vi "GetFileManagerDeviceConstants.vi"(9 "device":T2, 10 "key values":T13[](array[typedef]), 11 "config":T1) -> (3 "config out":T1)   [LabVIEW 2017]
uses:
  <vilib>/addons/InsightCM/MessageBus/Base/controls/SectionKeyValues.ctl
  <vilib>/addons/InsightCM/MessageBus/Base/controls/KeyValuePair.ctl
  <vilib>/addons/InsightCM/MessageBus/Base/controls/R2_Device.ctl
  <vilib>/addons/InsightCM/MessageBus/Base/controls/DeviceState.ctl
  <vilib>/addons/InsightCM/MessageBus/Base/controls/R2_DataGroup.ctl
  <vilib>/addons/InsightCM/MessageBus/Base/controls/OperatingState.ctl
  <vilib>/addons/InsightCM/MessageBus/Base/controls/Trigger.ctl
  <vilib>/addons/InsightCM/MessageBus/Base/controls/Condition.ctl
  <vilib>/addons/InsightCM/MessageBus/Base/controls/BurstModeTrigger.ctl
  <vilib>/addons/InsightCM/MessageBus/Base/controls/DeviceSensorGroup.ctl
  <vilib>/addons/InsightCM/MessageBus/Base/controls/Endpoint.ctl
  <vilib>/addons/InsightCM/MessageBus/Base/controls/WirelessChannel.ctl
  <vilib>/addons/InsightCM/Devices/Shared/Common/FileManager/controls/config.ctl
  <vilib>/addons/InsightCM/Utilities/PropertyHelpers/PropertyHelpers.lvlib
  <vilib>/addons/InsightCM/Devices/Shared/Common/FileManager/FileManager.lvlib
panel:
  out "backlog extra large files":bool
  out "backlog file batch size":i32
  out "backlog trend points":bool
  out "backlog stream trend points":bool
  out "clean up file folders interval (sec)":dbl
  out "backlog file interval (sec)":dbl
  out "max files in memory":i32
  out "min drive free space":i32
  out "manage drive interval (sec)":dbl
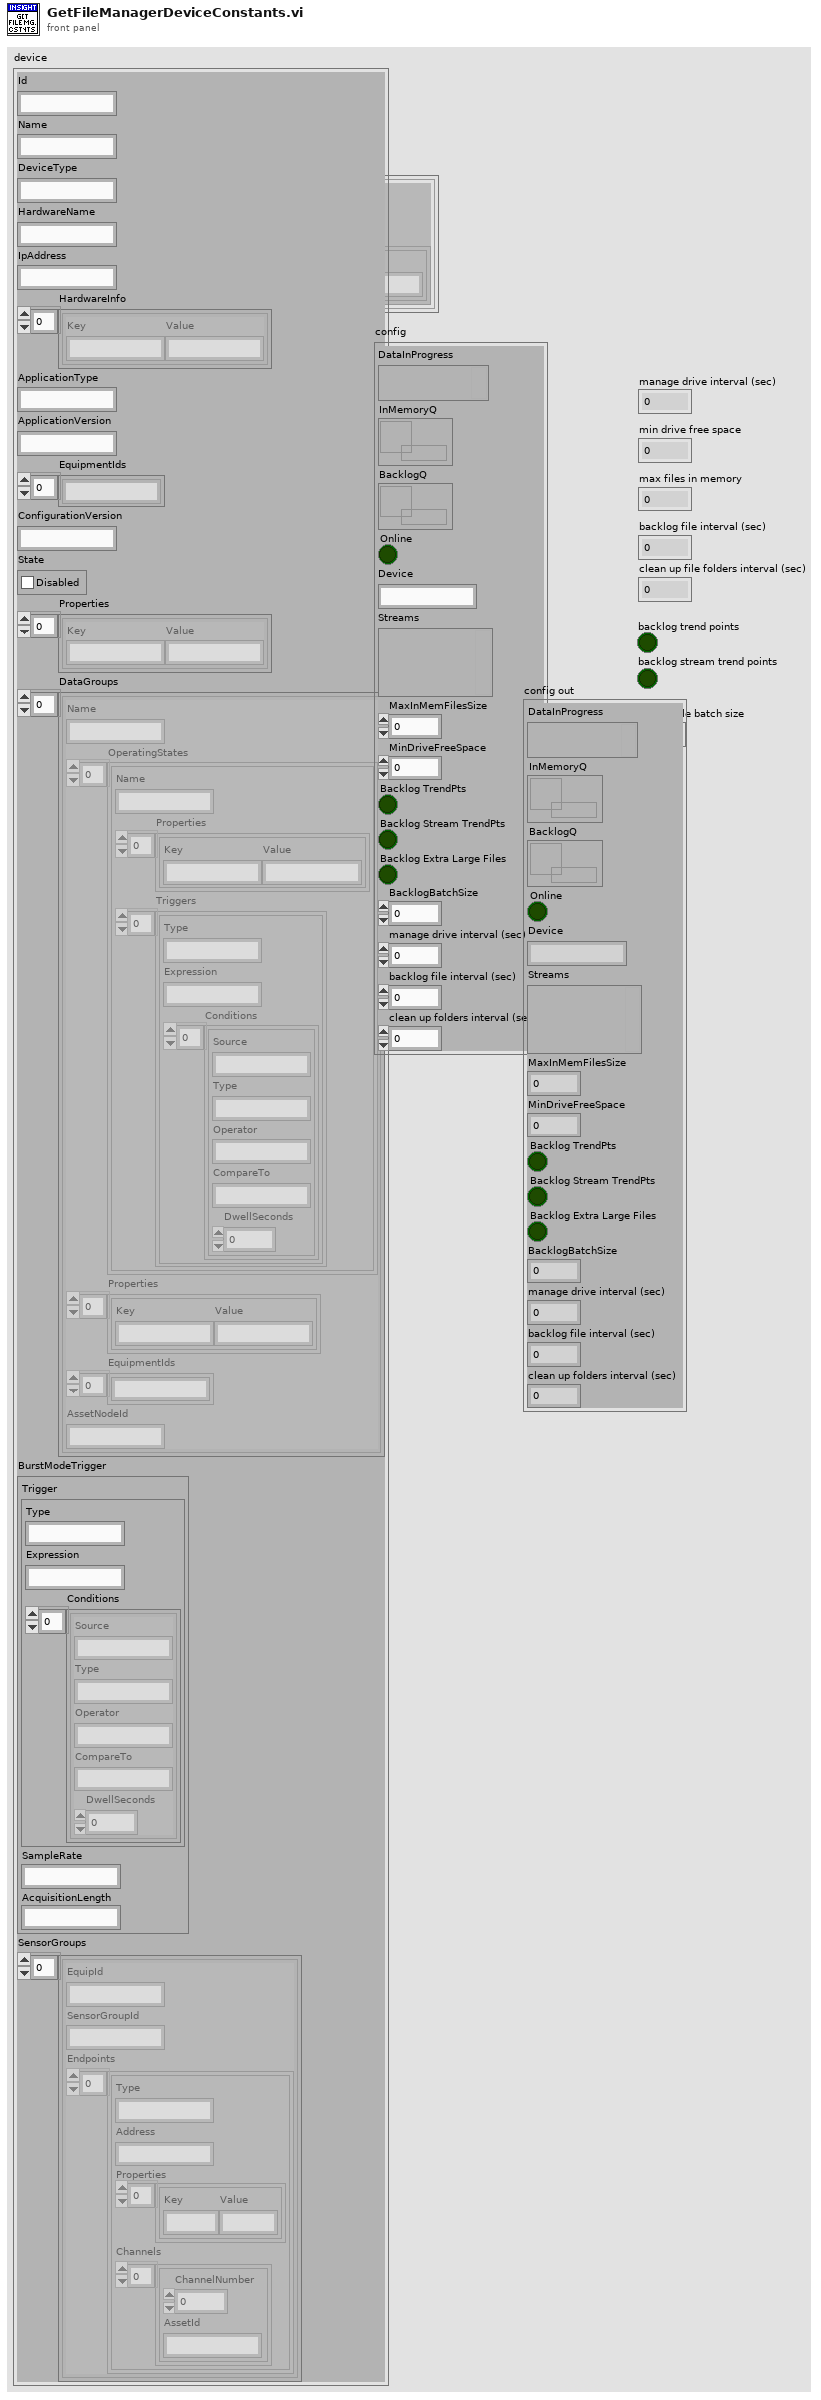
[diagram p1: front panel]
types:
  T1 = typedef "FileManager.lvlib/config.ctl" = cluster{"DataInProgress":variant, "InMemoryQ":refnum<queue>, "BacklogQ":refnum<queue>, "Online":bool, "Device":string, "Streams":variant, "MaxInMemFilesSize":i32, "MinDriveFreeSpace":i32, "Backlog TrendPts":bool, "Backlog Stream TrendPts":bool, "Backlog Extra Large Files":bool, "BacklogBatchSize":i32, "manage drive interval (sec)":dbl, "backlog file interval (sec)":dbl, "clean up folders interval (sec)":dbl}
  T2 = typedef "R2_Device.ctl" = cluster{"Id":string, "Name":string, "DeviceType":string, "HardwareName":string, "IpAddress":string, "HardwareInfo":T3[], "ApplicationType":string, "ApplicationVersion":string, "EquipmentIds":string[], "ConfigurationVersion":string, "State":T4, "Properties":T3[], "DataGroups":T5[], "BurstModeTrigger":T9, "SensorGroups":T10[]}
  T3 = typedef "KeyValuePair.ctl" = cluster{"Key":string, "Value":string}
  T4 = typedef "DeviceState.ctl" = cluster{"Disabled":bool}
  T5 = typedef "R2_DataGroup.ctl" = cluster{"Name":string, "OperatingStates":T6[], "Properties":T3[], "EquipmentIds":string[], "AssetNodeId":string}
  T6 = typedef "OperatingState.ctl" = cluster{"Name":string, "Properties":T3[], "Triggers":T7[]}
  T7 = typedef "Trigger.ctl" = cluster{"Type":string, "Expression":string, "Conditions":T8[]}
  T8 = typedef "Condition.ctl" = cluster{"Source":string, "Type":string, "Operator":string, "CompareTo":string, "DwellSeconds":dbl}
  T9 = typedef "BurstModeTrigger.ctl" = cluster{"Trigger":T7, "SampleRate":string, "AcquisitionLength":string}
  T10 = typedef "DeviceSensorGroup.ctl" = cluster{"EquipId":string, "SensorGroupId":string, "Endpoints":T11[]}
  T11 = typedef "Endpoint.ctl" = cluster{"Type":string, "Address":string, "Properties":T3[], "Channels":T12[]}
  T12 = typedef "WirelessChannel.ctl" = cluster{"ChannelNumber":i32, "AssetId":string}
  T13 = typedef "SectionKeyValues.ctl" = cluster{"Section":string, "KeyValues":T3[]}
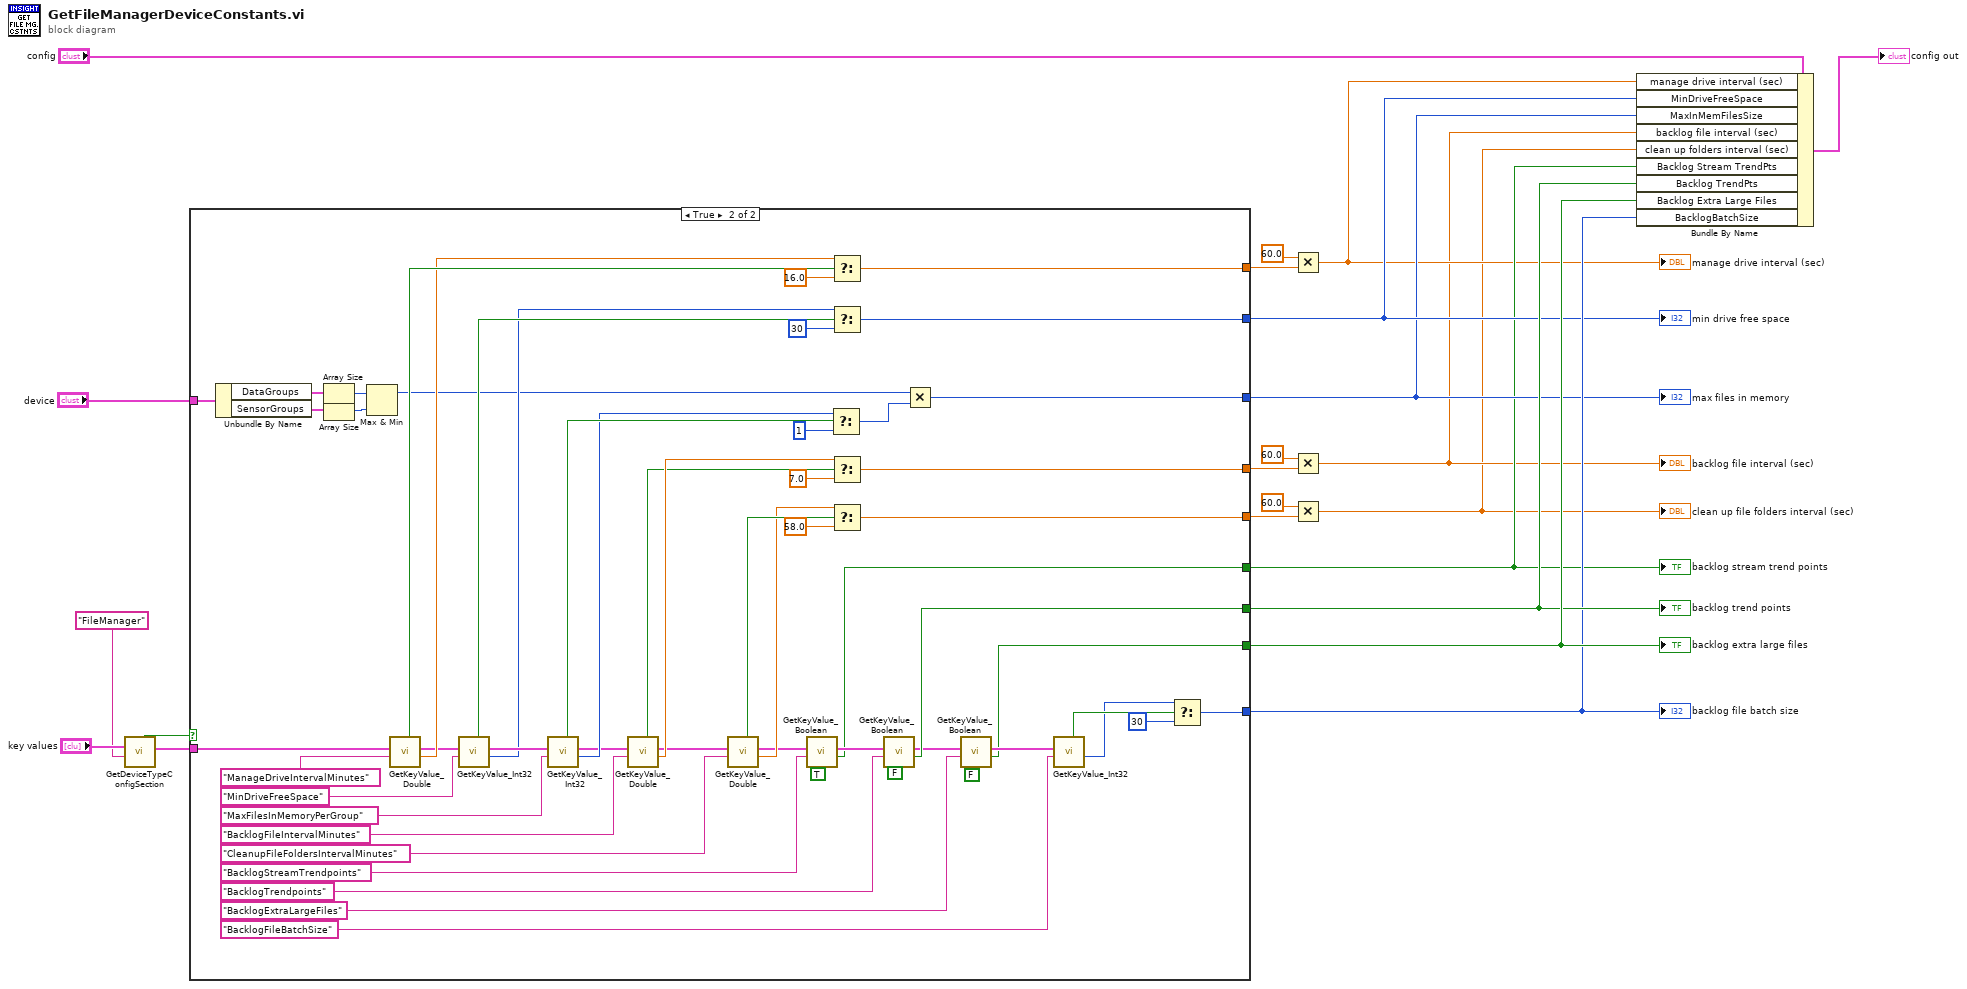
[diagram p0: block diagram]
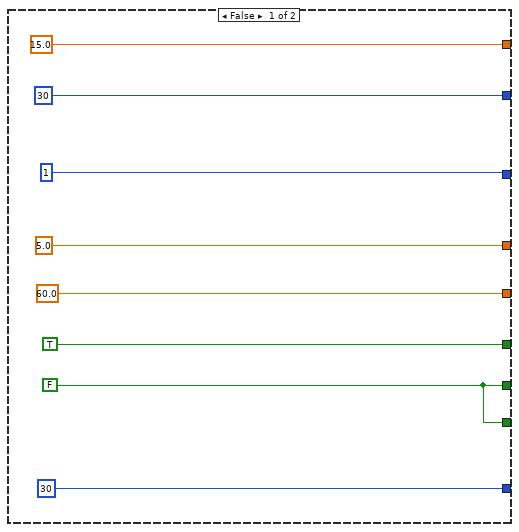
[diagram p2: hidden frame]
diagram:
  n1 = call <vilib>:"GetDeviceTypeConfigSection.vi"("key"="FileManager", "key values"="key values") -> ("key value pairs out"=w20:T3[], "found"=w21:bool)  [unwired: 8 in]
  n2 = case shown="True" w21 {
    tunnel: w20 -> [_ w85]
    tunnel: [15.0 ("f") w71] -> w18
    tunnel: [30 ("f") w70] -> w6
    tunnel: [1 ("f") w59] -> w5
    tunnel: [5.0 ("f") w66] -> w17
    tunnel: "device" -> [_ w62]
    tunnel: [60.0 ("f") w53] -> w12
    tunnel: [TRUE ("value") w40] -> w4
    tunnel: [w23 w42] -> w8
    tunnel: [30 ("f") w44] -> w7
    tunnel: [w23 w36] -> w9
    frame False {
      w23 = FALSE ("value")
    }
    frame True {
      n3 = Unbundle By Name(w62) -> ("DataGroups"=w61:T5[], "SensorGroups"=w34:T10[])
      n4 = Array Size(array=w61) -> (size(s)=w32:i32)
      n5 = Array Size(array=w34) -> (size(s)=w33:i32)
      n6 = Max & Min(x=w32, y=w33) -> (max(x,y)=w31:i32)  [unwired: 1 out]
      n7 = call <vilib>:"GetKeyValue_Double.vi"("key"="ManageDriveIntervalMinutes" ("Key"), "key value pairs"=w85) -> ("value"=w83:dbl, "key value pairs out"=w81:T3[], "found"=w84:bool)  [unwired: 7 in]
      n8 = call <vilib>:"GetKeyValue_Int32.vi"("key"="MinDriveFreeSpace" ("Key"), "key value pairs"=w81) -> ("value"=w76:i32, "key value pairs out"=w80:T3[], "found"=w78:bool)  [unwired: 7 in]
      n9 = call <vilib>:"GetKeyValue_Int32.vi"("key"="MaxFilesInMemoryPerGroup", "key value pairs"=w80) -> ("value"=w75:i32, "key value pairs out"=w67:T3[], "found"=w77:bool)  [unwired: 7 in]
      n10 = call <vilib>:"GetKeyValue_Double.vi"("key"="BacklogFileIntervalMinutes" ("Key"), "key value pairs"=w67) -> ("value"=w64:dbl, "key value pairs out"=w55:T3[], "found"=w63:bool)  [unwired: 7 in]
      n11 = call <vilib>:"GetKeyValue_Double.vi"("key"="CleanupFileFoldersIntervalMinutes" ("Key"), "key value pairs"=w55) -> ("value"=w57:dbl, "key value pairs out"=w52:T3[], "found"=w58:bool)  [unwired: 7 in]
      n12 = call <vilib>:"GetKeyValue_Boolean.vi"("default value"=TRUE, "key"="BacklogStreamTrendpoints", "key value pairs"=w52) -> ("value"=w40:bool, "key value pairs out"=w50:T3[])  [unwired: 6 in, 1 out]
      n13 = Select(t=w75, s=w77, f=1) -> (s? t:f=w60:i32)
      n14 = Select(t=w83, s=w84, f=16.0) -> (s? t:f=w71:dbl)
      n15 = Select(t=w76, s=w78, f=30) -> (s? t:f=w70:i32)
      n16 = Select(t=w64, s=w63, f=7.0) -> (s? t:f=w66:dbl)
      n17 = Select(t=w57, s=w58, f=58.0) -> (s? t:f=w53:dbl)
      n18 = call <vilib>:"GetKeyValue_Boolean.vi"("default value"=FALSE, "key"="BacklogTrendpoints", "key value pairs"=w50) -> ("value"=w42:bool, "key value pairs out"=w39:T3[])  [unwired: 6 in, 1 out]
      n19 = Multiply(x=w31, y=w60) -> (x*y=w59:i32)
      n20 = call <vilib>:"GetKeyValue_Boolean.vi"("default value"=FALSE, "key"="BacklogExtraLargeFiles", "key value pairs"=w39) -> ("value"=w36:bool, "key value pairs out"=w38:T3[])  [unwired: 6 in, 1 out]
      n21 = call <vilib>:"GetKeyValue_Int32.vi"("key"="BacklogFileBatchSize", "key value pairs"=w38) -> ("value"=w46:i32, "found"=w47:bool)  [unwired: 7 in, 1 out]
      n22 = Select(t=w46, s=w47, f=30) -> (s? t:f=w44:i32)
    }
  }
  "min drive free space" <- w6
  "max files in memory" <- w5
  "backlog stream trend points" <- w4
  "backlog trend points" <- w8
  "backlog file batch size" <- w7
  "backlog extra large files" <- w9
  n23 = Multiply(x=60.0, y=w18) -> (x*y=w3:dbl)
  "manage drive interval (sec)" <- w3
  n24 = Multiply(x=60.0, y=w17) -> (x*y=w2:dbl)
  "backlog file interval (sec)" <- w2
  n25 = Multiply(x=60.0, y=w12) -> (x*y=w1:dbl)
  "clean up file folders interval (sec)" <- w1
  n26 = Bundle By Name(cluster="config", "manage drive interval (sec)"=w3, "MinDriveFreeSpace"=w6, "MaxInMemFilesSize"=w5, "backlog file interval (sec)"=w2, "clean up folders interval (sec)"=w1, "Backlog Stream TrendPts"=w4, "Backlog TrendPts"=w8, "Backlog Extra Large Files"=w9, "BacklogBatchSize"=w7) -> (→"config out":T1)
